vi "validate email address.vi"(11 "Email address in":string="hm328@exeter.ac.uk") -> (2 "Valid?":bool, 3 "Email address out":string)   [LabVIEW 2014]
uses:
  <vilib>/regexp/Match Regular Expression.xnode
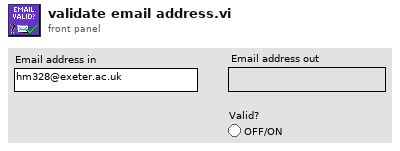
[diagram p1: front panel]
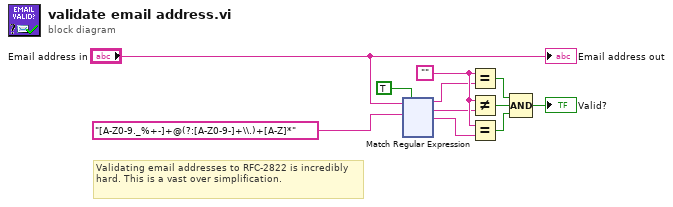
[diagram p0: block diagram]
diagram:
  w6 = ""
  # "Validating email addresses to RFC-2822 is incredibly hard. This is a vast over simplification."
  n1 = xnode "Match Regular Expression"("input string"="Email address in", "regular expression"="[A-Z0-9._%+-]+@(?:[A-Z0-9-]+\\.)+[A-Z]*", "ignore case? (F)"=TRUE) -> ("before match"=w3:string, "whole match"=w5:string, "after match"=w4:string)  [unwired: 3 in, 2 out]
  n2 = Equal?(x=w6, y=w3) -> (x = y?=w7:bool)
  n3 = Not Equal?(x=w6, y=w5) -> (x != y?=w8:bool)
  n4 = Equal?(x=w6, y=w4) -> (x = y?=w9:bool)
  n5 = Compound Arithmetic op=AND(w7, w8, w9) -> (→"Valid?":bool)
  "Email address out" <- "Email address in"
